vi "Generate Sine Wave for Digital Audio - Crosstalk.vi"(5 "interferrer channel":i32, 6 "number of channels":i32, 7 "output level units":T1, 9 "phase":dbl, 10 "amplitude":dbl=0.5, 11 "frequency":dbl=0.5) -> (3 "signals":T2(array[cluster]))   [LabVIEW 2023]
uses:
  controls/digital output level units.ctl
  controls/audio controls.lvlib
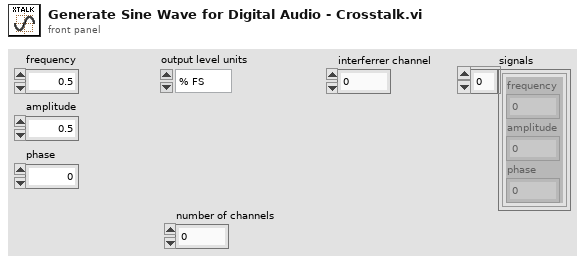
[diagram p1: front panel]
types:
  T1 = typedef "audio controls.lvlib/digital output level units.ctl" = enum32{"% FS", "dBFS", "V"}
  T2 = cluster{"frequency":dbl, "amplitude":dbl, "phase":dbl}[]
  T3 = cluster{"frequency":dbl, "amplitude":dbl, "phase":dbl}
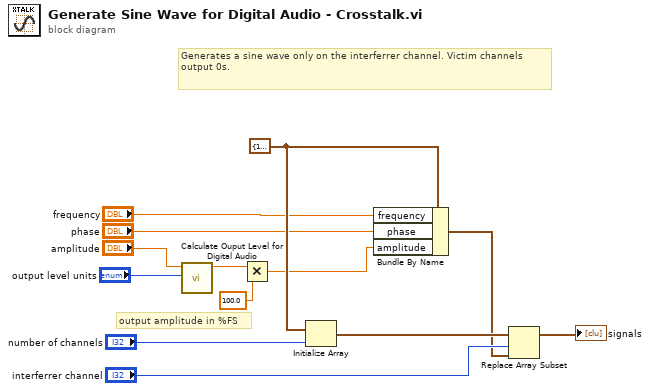
[diagram p0: block diagram]
diagram:
  w10 = T3 {"frequency"=1000.0, "amplitude"=0.0, "phase"=0.0} ("sine wave")
  # "output amplitude in %FS"
  # "Generates a sine wave only on the interferrer channel. Victim channels output 0s."
  n1 = call "Calculate Ouput Level for Digital Audio.vi"("digital output level units"="output level units", "output level"="amplitude") -> ("gain"=w3:dbl)  [unwired: 8 in, 1 out]
  n2 = Multiply(x=w3, y=100.0) -> (x*y=w1:dbl)
  n3 = Initialize Array(w10, "number of channels") -> (w12:T2)
  n4 = Bundle By Name(cluster=w10, "frequency"="frequency", "phase"="phase", "amplitude"=w1) -> (w7:T3)
  n5 = Replace Array Subset(array=w12, new element=w7, index="interferrer channel") -> (→"signals":T2)
